vi "LeerBD.vi"(8 "error in (no error)":errorcluster) -> (0 "error out":errorcluster, 2 "BD":T1={"niv_presion_son_ref"=97.0, "min_rango_ref"=97.0, "max_rango_ref"=97.0, "Incertidumbre"=[], "Tol +"=[], "Tol -"=[]}, 3 "Prueba08 out":refnum<class "Prueba08.lvclass">)   [LabVIEW 2019, in "Prueba08.lvclass"]
uses:
  Prueba08.lvclass
  BD.ctl
  Base de Datos/SQLiteConnector/SQLiteConnection.lvclass
  Base de Datos/Base de Datos.lvclass
panel:
  in  "Tipo Equipo":enum16{"Sonometro", "Calibrador", "Dosimetro"}(ring)
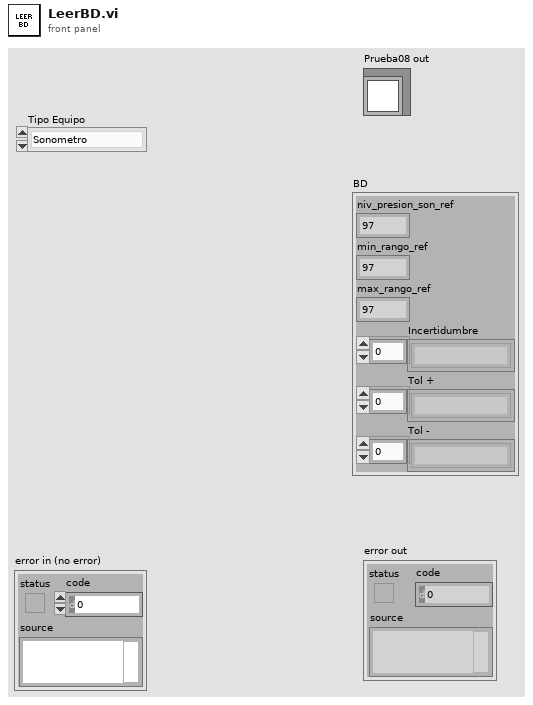
[diagram p1: front panel]
types:
  T1 = typedef "Prueba08.lvclass/BD.ctl" = cluster{"niv_presion_son_ref":dbl, "min_rango_ref":dbl, "max_rango_ref":dbl, "Incertidumbre":string[], "Tol +":string[], "Tol -":string[]}
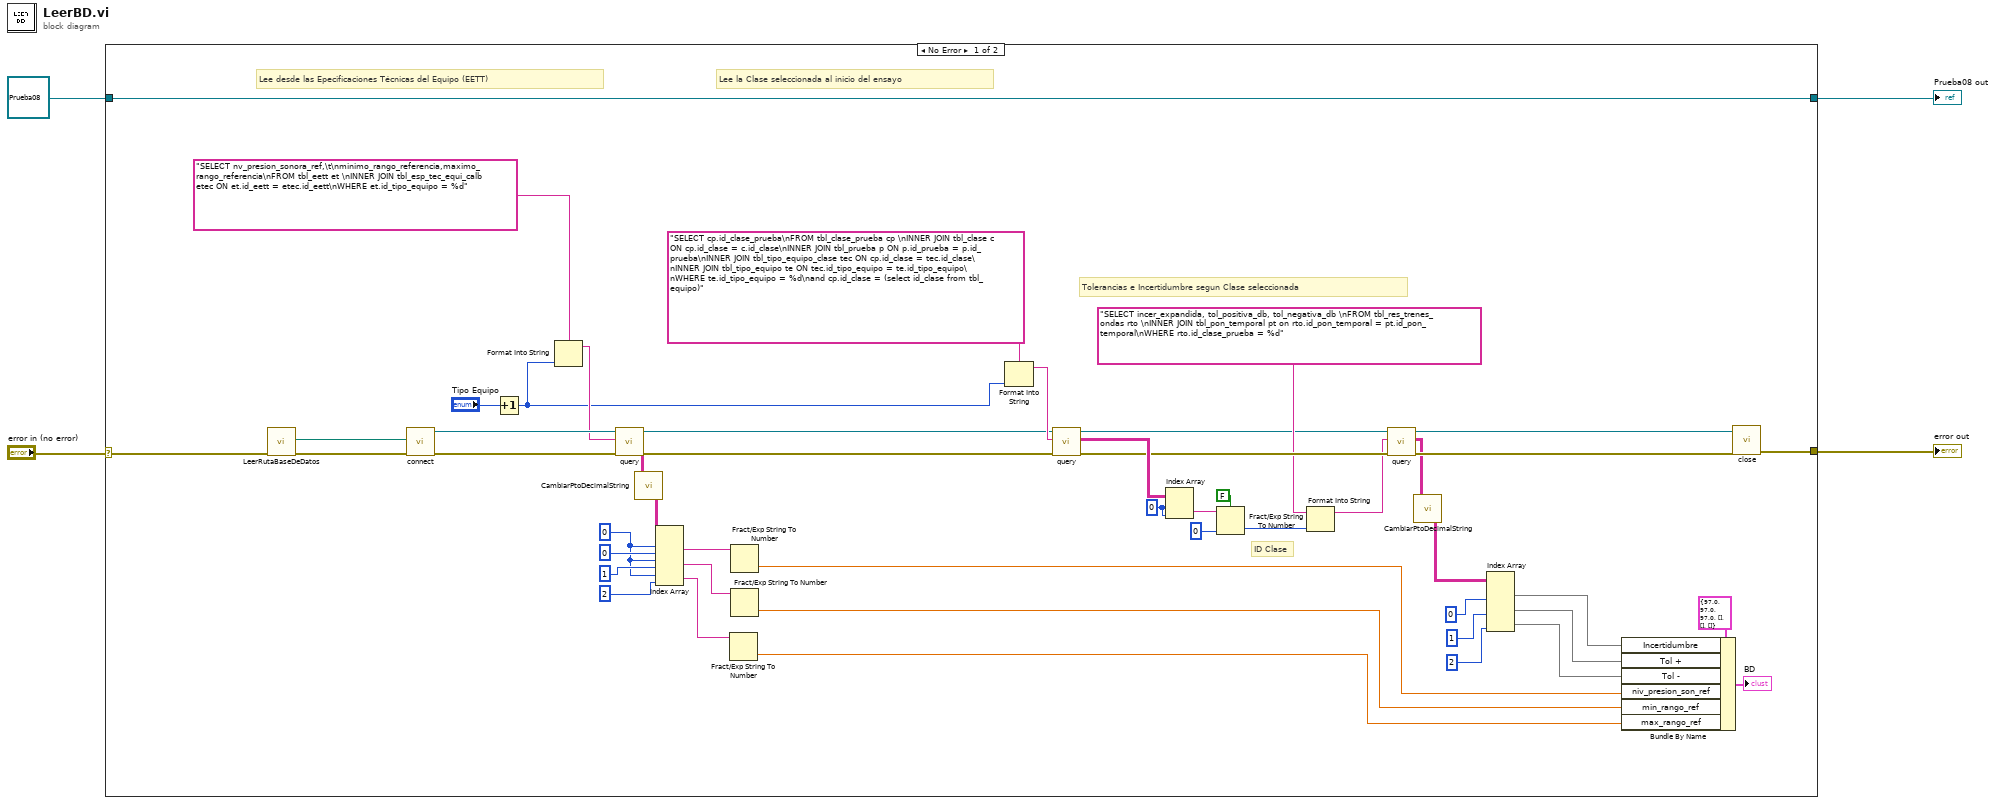
[diagram p0: block diagram]
diagram:
  n1 = case shown="No Error" "error in (no error)" {
    selector: "error in (no error)" -> [w45 w55]
    tunnel: [w32 w55] -> w3
    tunnel: [w53 w54] -> w1
    tunnel: refnum<class "Prueba08.lvclass"> refnum ("Prueba02 in") -> [w53 w54]
    frame No Error {
      w38 = 0 ("index (row)")
      w13 = 0 ("index (row)")
      # "Tolerancias e Incertidumbre segun Clase seleccionada"
      # "ID Clase"
      # "Lee la Clase seleccionada al inicio del ensayo"
      # "Lee desde las Epecificaciones Técnicas del Equipo (EETT)"
      n2 = call "LeerRutaBaseDeDatos.vi"("error in (no error)"=w45) -> ("error out"=w48:errorcluster, "Database Path"=w47:path)  [unwired: 9 in]
      n3 = call "connect.vi"("error in (no error)"=w48, "Database Path"=w47) -> ("error out"=w50:errorcluster, "object out"=w51:refnum<class "SQLiteConnection.lvclass">)  [unwired: 8 in]
      n4 = Increment(x="Tipo Equipo") -> (x+1=w27:enum16{"Sonometro", "Calibrador", "Dosimetro"})
      n5 = Format Into String(format string="SELECT nv_presion_sonora_ref,\t\nminimo_rango_referencia,maximo_rango_referencia\nFROM tbl_eett et \nINNER JOIN tbl_esp_tec_equi_calb etec ON et.id_eett = etec.id_eett\nWHERE et.id_tipo_equipo = %d", w27) -> (resulting string=w49:string)  [unwired: 2 in, 1 out]
      n6 = call "query.vi"("error in (no error)"=w50, "SQL Statement"=w49, "object in"=w51) -> ("error out"=w39:errorcluster, "result"=w16:string[][], "object out"=w40:refnum<class "SQLiteConnection.lvclass">)  [unwired: 5 in, 1 out]
      n7 = call "CambiarPtoDecimalString.vi"("result"=w16) -> ("result out"=w5:string[][])
      n8 = Index Array(array=w5, index (row) #1=w13, index (col) #1=0 ("disabled index (col)"), index (row) #2=w13, index (col) #2=1 ("disabled index (col)"), index (row) #3=w13, index (col) #3=2 ("disabled index (col)")) -> (element #1=w43:string, element #2=w21:string, element #3=w11:string)
      n9 = Fract/Exp String To Number(string=w11) -> (number=w10:dbl)  [unwired: 3 in, 1 out]
      n10 = Fract/Exp String To Number(string=w43) -> (number=w23:dbl)  [unwired: 3 in, 1 out]
      n11 = Fract/Exp String To Number(string=w21) -> (number=w20:dbl)  [unwired: 3 in, 1 out]
      n12 = Format Into String(format string="SELECT cp.id_clase_prueba\nFROM tbl_clase_prueba cp \nINNER JOIN tbl_clase c ON cp.id_clase = c.id_clase\nINNER JOIN tbl_prueba p ON p.id_prueba = p.id_prueba\nINNER JOIN tbl_tipo_equipo_clase tec ON cp.id_clase = tec.id_clase\nINNER JOIN tbl_tipo_equipo te ON tec.id_tipo_equipo = te.id_tipo_equipo\nWHERE te.id_tipo_equipo = %d\nand cp.id_clase = (select id_clase from tbl_equipo)", w27) -> (resulting string=w41:string)  [unwired: 2 in, 1 out]
      n13 = call "query.vi"("error in (no error)"=w39, "SQL Statement"=w41, "object in"=w40) -> ("error out"=w33:errorcluster, "result"=w34:string[][], "object out"=w29:refnum<class "SQLiteConnection.lvclass">)  [unwired: 5 in, 1 out]
      n14 = Index Array(array=w34, index (row)=w38, index (col)=w38) -> (element=w36:string)
      n15 = Fract/Exp String To Number(use system decimal point (T)=FALSE, string=w36, default (0 dbl)=0 ("index (row)")) -> (number=w24:i32)  [unwired: 1 in, 1 out]
      n16 = Format Into String(format string="SELECT incer_expandida, tol_positiva_db, tol_negativa_db \nFROM tbl_res_trenes_ondas rto \nINNER JOIN tbl_pon_temporal pt on rto.id_pon_temporal = pt.id_pon_temporal\nWHERE rto.id_clase_prueba = %d", w24) -> (resulting string=w28:string)  [unwired: 2 in, 1 out]
      n17 = call "query.vi"("error in (no error)"=w33, "SQL Statement"=w28, "object in"=w29) -> ("error out"=w30:errorcluster, "result"=w26:string[][], "object out"=w25:refnum<class "SQLiteConnection.lvclass">)  [unwired: 5 in, 1 out]
      n18 = call "CambiarPtoDecimalString.vi"("result"=w26) -> ("result out"=w6:string[][])
      n19 = Index Array(array=w6, index (col) #1=0 ("disabled index (col)"), index (col) #2=1 ("disabled index (col)"), index (col) #3=2 ("disabled index (col)")) -> (element #1=w9:string[], element #2=w8:string[], element #3=w7:string[])  [unwired: 3 in]
      n20 = Bundle By Name(cluster=T1 {"niv_presion_son_ref"=97.0, "min_rango_ref"=97.0, "max_rango_ref"=97.0, "Incertidumbre"=[], "Tol +"=[], "Tol -"=[]} ("BD"), "Incertidumbre"=w9, "Tol +"=w8, "Tol -"=w7, "niv_presion_son_ref"=w23, "min_rango_ref"=w20, "max_rango_ref"=w10) -> (→"BD":T1)
      n21 = call-dynamic "close.vi"("error in (no error)"=w30, "object in"=w25) -> ("error out"=w32:errorcluster)  [unwired: 8 in, 1 out]
    }
    frame Error {
    }
  }
  "error out" <- w3
  "Prueba08 out" <- w1
